vi "brc_daq_start_DAQ.vi"(2 "rawValue":u8, 5 "error in (no error)":errorcluster, 6 "mHandle":i32) -> (19 "error out":errorcluster)   [LabVIEW 2019, in "BRC-DAQ.lvlib"]
uses:
  BRC-DAQ.lvlib
panel:
  out "return_value":i32
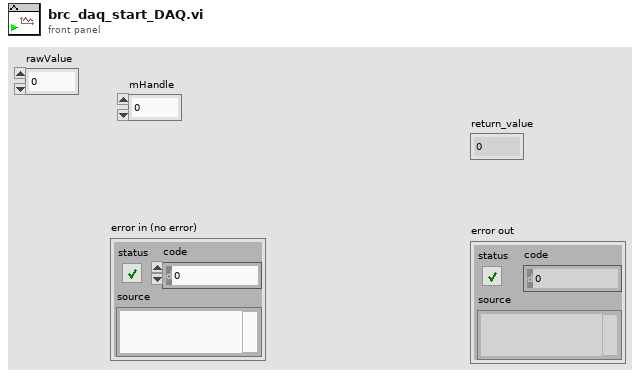
[diagram p1: front panel]
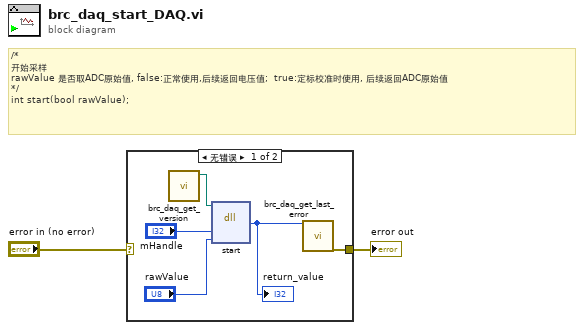
[diagram p0: block diagram]
diagram:
  # "/*\n开始采样\nrawValue 是否取ADC原始值, false:正常使用,后续返回电压值;  true:定标校准时使用, 后续返回ADC原始值\n*/\nint start(bool rawValue);"
  n1 = case shown="无错误" "error in (no error)" {
    selector: "error in (no error)" -> [_ w8]
    tunnel: [w6 w8] -> w2
    frame No Error {
      n2 = call "brc_daq_get_version.vi"() -> ("dll path"=w3:path)  [unwired: 11 in]
      n3 = dll-call lib="E:/01 BRC project/04BRC-daq/04 Drive/DAQ-x64/DLL/brc_daq_sdk.dll" fn="start"(path in=w3, "mHandle"="mHandle", "rawValue"="rawValue") -> ("return type"=w7:i32)  [unwired: 4 in, 2 out]
      "return_value" <- w7
      n4 = call "brc_daq_get_last_error.vi"("return_value"=w7) -> ("error out"=w6:errorcluster)  [unwired: 18 in]
    }
    frame Error {
    }
  }
  "error out" <- w2
